vi "CleanUp.vi"(8 "error in (no error)":errorcluster, 11 "pressureSensor in":refnum<class "pressureSensor.lvclass">) -> (0 "error out":errorcluster, 3 "pressureSensor out":refnum<class "pressureSensor.lvclass">)   [LabVIEW 2020, in "RPI.SenseHat.Sensors.lvlib" / "pressureSensor.lvclass"]
uses:
  pressureSensor.lvclass
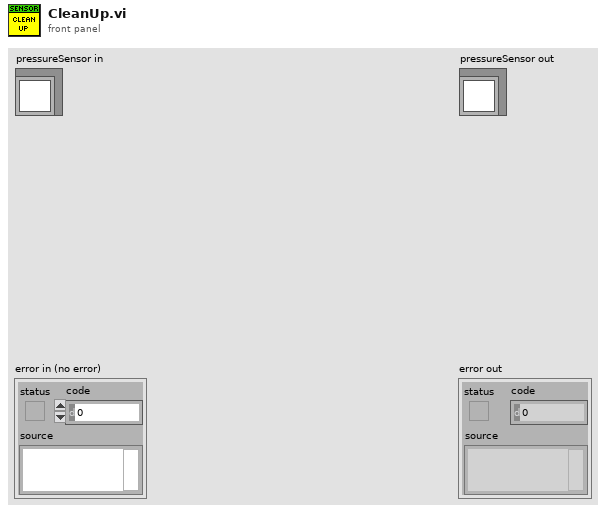
[diagram p1: front panel]
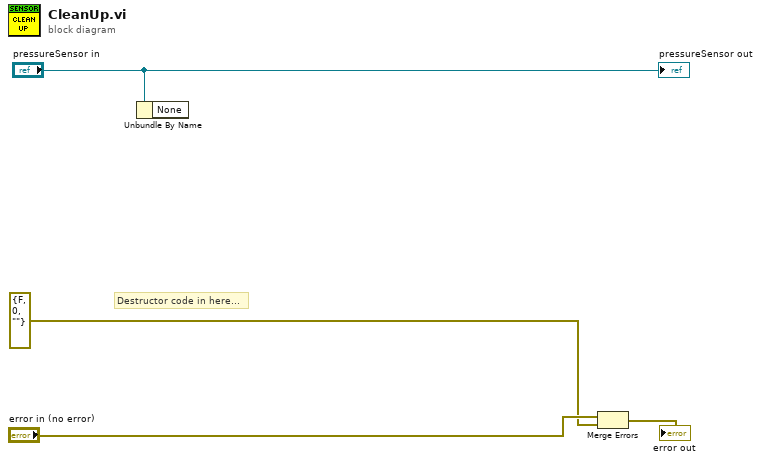
[diagram p0: block diagram]
diagram:
  # "Destructor code in here..."
  n1 = Unbundle By Name("pressureSensor in") -> ()  [unwired: 1 out]
  n2 = Merge Errors("error in (no error)", errorcluster {"status"=FALSE, "code"=0, "source"=""} ("error in (no error)")) -> (→"error out":errorcluster)
  "pressureSensor out" <- "pressureSensor in"
